vi "tip_transform.vi"(11 "Trace record":sgl[][](array[numeric])) -> (3 "To tip transform":T1)   [LabVIEW 2013]
uses:
  <vilib>/Analysis/Matrix/Datatypes/RealMatrix.ctl
  pose_source.ctl
  <vilib>/Analysis/baseanly.llb/Real A x B.vi
  initialization/micron_globals.vi
  <vilib>/Analysis/Matrix/Numeric/Conversions/Array To Matrix - RA.vi
  <vilib>/Analysis/Matrix/NI_Matrix.lvlib
  <vilib>/Analysis/NI_AALBase.lvlib
panel:
  # "Given a trace data record, compute the transform matrix to convert into tool tip coordinates."
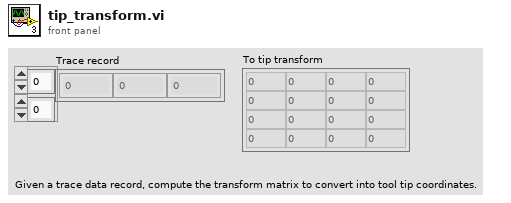
[diagram p1: front panel]
types:
  T1 = typedef "NI_Matrix.lvlib/RealMatrix.ctl" = dbl[][]
  T2 = typedef "pose_source.ctl" = enum16{"Output", "Handle", "Handle KF", "Goal", "Absolute"}
  T3 = typedef "Micron params.ctl" = cluster{"Stimulus":T4, "Goal Filter A":T6, "Mode controls":T7, "Manipulator type":enum16{"Current piezo", "Voltage piezo"}, "Manipulator calibration":T8, "Network":T10, "Goal Filter B":T6, "Cancellation":T11, "Transition time":sgl, "Estimation":T13}
  T4 = typedef "stimulus.ctl" = cluster{"Type":enum16{"Off", "Step", "Sine", "Triangle", "Arbitrary"}, "Phase":dbl, "Amplitude":sgl[], "Injection point":T5, "Closed loop":bool, "Offset":sgl[], "Tip -> world":bool, "Frequency":dbl, "Length":dbl}
  T5 = typedef "injection_point.ctl" = enum16{"Total pose", "V limiter", "Goal ", "Link position", "KF link position", "Inverse kin", "Link goal", "Link error", "Controller", "Output", "Drive", "Light"}
  T6 = typedef "goal_loop_parms.ctl" = cluster{"Speedup max":sgl, "Speedup thresh":sgl, "Speedup nonlin":sgl, "Filters":cluster{"Lower Fc":sgl, "Lower Q":sgl, "Scale factor":sgl, "Upper Fc":sgl, "Upper Q":sgl, "V limit":sgl, "V limit range":sgl}[]}
  T7 = typedef "mode_conrols.ctl" = cluster{"Hold":bool, "Cancellation":bool, "Goal filter":bool, "Trigger":bool}
  T8 = typedef "manipulator_cal.ctl" = cluster{"Tool offsets":sgl[][], "Tip light calibration":T9, "Handle light calibration":T9, "Base pivots":sgl[][], "Output pivots":sgl[][], "Length center":sgl, "Workspace height":sgl[], "Workspace diameter":sgl[], "Linearization":sgl[][], "Stack travel":sgl, "Saturation pos":sgl, "Inverse filters":cluster{"filter structure":enum32{"IIR 2nd Order", "IIR 4th Order"}, "Reverse Coefficients":dbl[], "Forward Coefficients":dbl[]}[]}
  T9 = typedef "probe_calibration.ctl" = sgl[][]
  T10 = typedef "network_params.ctl" = cluster{"Remote Host":string, "Send Status":bool, "Send Port":u16, "Recv Commands":bool, "Recv Port":u16}
  T11 = typedef "sq_control_params.ctl" = cluster{"KP":T12, "KI":sgl, "KD":T12, "Max vel":sgl, "Max acc":sgl, "Int error limit":sgl, "RCM gain":sgl, "Bypass":bool, "Degraded gain":sgl}
  T12 = typedef "decoupled_gain.ctl" = cluster{"XY":sgl, "Rxy":sgl, "Z":sgl, "Rz":sgl}
  T13 = typedef "estimation_controls.ctl" = cluster{"Link":cluster{"Measure noise":dbl[], "Process noise":dbl[], "Alt process noise":dbl[], "Alt turnoff cycles":i32, "Innovation limit":dbl[], "Residue threshold":dbl, "Enable":bool}, "Handle":cluster{"Measure noise":dbl[], "Process noise":dbl[], "State limits":dbl[], "Innovation limit":dbl[], "Prediction Lookahead":sgl, "Enable":bool}}
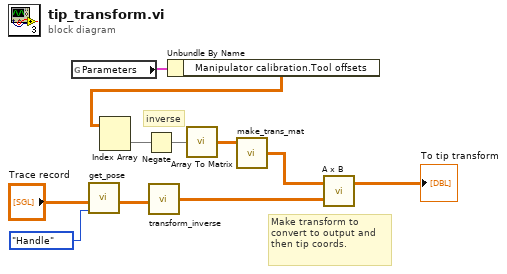
[diagram p0: block diagram]
diagram:
  # "inverse"
  # "Make transform to convert to output and then tip coords."
  n1 = global read "micron_globals.vi" "Parameters"() -> (w5:T3)
  n2 = call "get_pose.vi"("Selector"=pose_source."Handle", "Input Trace"="Trace record") -> ("Pose"=w9:T1)  [unwired: 9 in]
  n3 = call "transform_inverse.vi"("Transform"=w9) -> ("Inverse transform"=w6:T1)
  n4 = Unbundle By Name(w5) -> ("Manipulator calibration.Tool offsets"=w10:sgl[][])
  n5 = Index Array(array=w10) -> (element=w11:sgl[])  [unwired: 2 in]
  n6 = Negate(x=w11) -> (-x=w4:sgl[])
  n7 = call-poly <vilib>:"Array To Matrix.vi"("Real 1D Array"=w4) -> ("Real Matrix (Column Vector)"=w3:T1)
  n8 = call "make_trans_mat.vi"("Translation"=w3) -> ("Transform"=w2:T1)  [unwired: 1 in, 3 out]
  n9 = call-poly <vilib>:"A x B.vi"("B"=w6, "A"=w2) -> ("A x B"=→"To tip transform":T1)  [unwired: 1 out]
